vi "Elevator_Hopper_Manual.vi"(0 "Elevator_Control":T1={"DeviceStatus"={"status"=FALSE, "code"=0, "source"=""}, "Type"=enum."PWM", "PWM"={"PWM Channel"=enum."Invalid", "DeadBand"={"Name"="", "maxPositivePwm"=0, "minPositivePwm"=0, "centerPwm"=0, "maxNegativePwm"=0, "minNegativePwm"=0, "angularRange"=0}}, "CAN"={"Device Number"=0, "SetOutput VI Ref"=variant(enum8{"Percent VBus", "Current", "Speed", "Position", "Voltage"} enum."Percent VBus"), "GetOutput VI Ref"=variant(refnum<k1> refnum), "Enable VI Ref"=variant(dbl 12.0), "Disable VI Ref"=variant(enum8{"Percent VBus", "Speed", "Position", "Slave", "Unchanged / Invalid"} enum."Percent VBus"), "Data"=variant}, "Invert"=FALSE, "DIO PWM"={"PWM \"Enable\" Channel"=enum."Invalid", "DIOChannel"=enum."Invalid", "PWM Rate"=0.0}}, 1 "Hopper_Control":T1={"DeviceStatus"={"status"=FALSE, "code"=0, "source"=""}, "Type"=enum."PWM", "PWM"={"PWM Channel"=enum."Invalid", "DeadBand"={"Name"="", "maxPositivePwm"=0, "minPositivePwm"=0, "centerPwm"=0, "maxNegativePwm"=0, "minNegativePwm"=0, "angularRange"=0}}, "CAN"={"Device Number"=0, "SetOutput VI Ref"=variant(enum8{"Percent VBus", "Current", "Speed", "Position", "Voltage"} enum."Percent VBus"), "GetOutput VI Ref"=variant(refnum<k1> refnum), "Enable VI Ref"=variant(dbl 12.0), "Disable VI Ref"=variant(enum8{"Percent VBus", "Speed", "Position", "Slave", "Unchanged / Invalid"} enum."Percent VBus"), "Data"=variant}, "Invert"=FALSE, "DIO PWM"={"PWM \"Enable\" Channel"=enum."Invalid", "DIOChannel"=enum."Invalid", "PWM Rate"=0.0}}, 2 "Ball at Top":bool, 3 "Shoot":bool, 5 "Elevator_up":bool, 7 "Distance_to_target (in)":dbl, 9 "Elevator_Down":bool, 11 "Hopper Forwards":bool, 12 "Hopper Backwards":bool, 13 "Intake":bool) -> ()   [LabVIEW 2019]
uses:
  <vilib>/Rock Robotics/WPI/MotorControl/WPI_MotorControlDeviceRef.ctl
  <vilib>/Rock Robotics/WPI/MotorControl/WPI_MotorControlType.ctl
  <vilib>/Rock Robotics/SystemInterfaces/DIO/FPGA_DIOPWMChannel.ctl
  <vilib>/Rock Robotics/WPI/PWM/WPI_PWMDeadband.ctl
  <vilib>/Rock Robotics/SystemInterfaces/DIO/FPGA_DIOChannel.ctl
  ArgosLib/Signal Processing/TypeDefs/EdgeDetector_Type.ctl
  ArgosLib/ArgosLib.lvlib
panel:
  in  "Off":dbl[](array[numeric])=[0.0, 0.0, 0.0, 0.0, 0.0, 0.0]
  in  "Elevator Speeds down":dbl[](array[numeric])=[-0.8, -0.8, -0.8, -0.8, -0.8, -0.8]
  in  "Distances (in)":dbl[](array[numeric])=[51.5, 57.5, 120.0, 240.0, 360.0, 480.0]
  in  "Elevator Speeds":dbl[](array[numeric])=[1.0, 1.0, 0.6, 0.5, 0.4, 0.4]
  in  "Bakwards_Hopper":dbl=-0.5
  in  "Forwards_Hopper":dbl=0.7
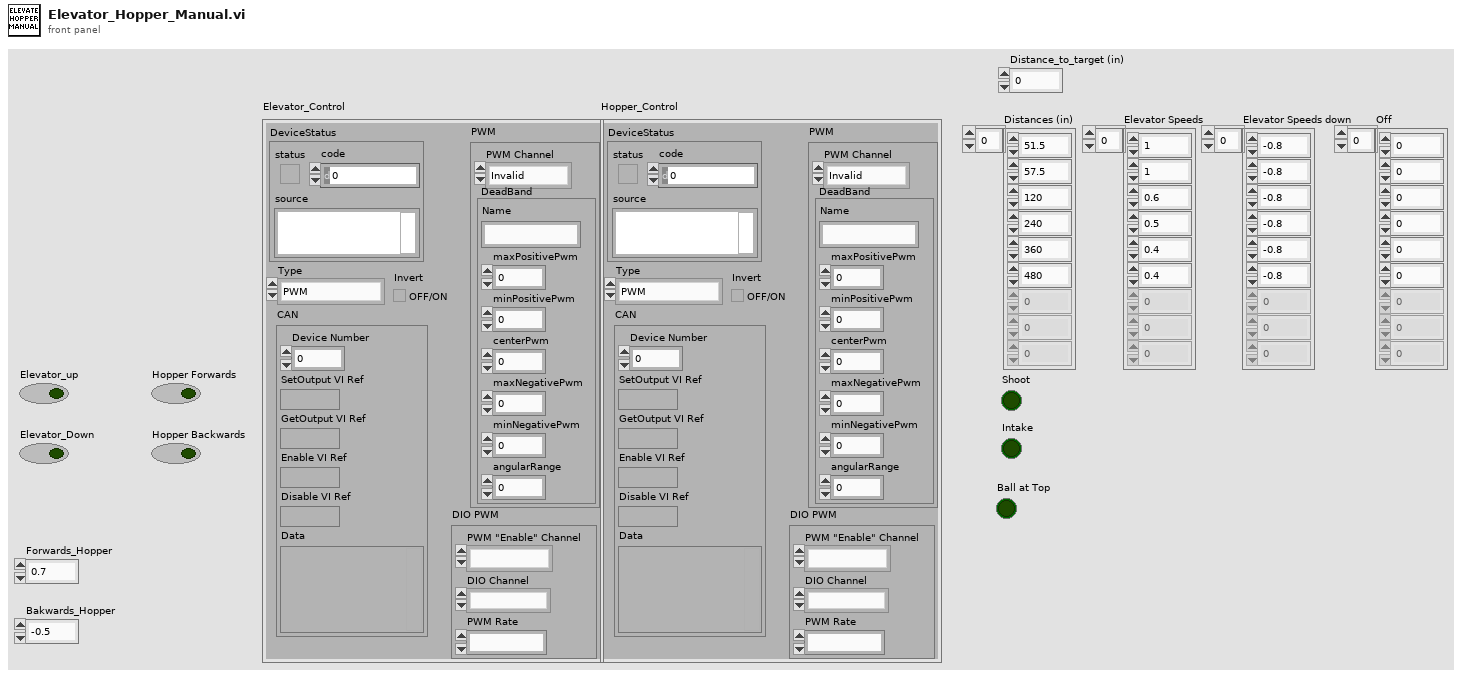
[diagram p1: front panel]
types:
  T1 = typedef "WPI_MotorControlDeviceRef.ctl" = cluster{"DeviceStatus":errorcluster, "Type":T2, "PWM":cluster{"PWM Channel":T3, "DeadBand":T4}, "CAN":cluster{"Device Number":u8, "SetOutput VI Ref":variant, "GetOutput VI Ref":variant, "Enable VI Ref":variant, "Disable VI Ref":variant, "Data":variant}, "Invert":bool, "DIO PWM":cluster{"PWM \"Enable\" Channel":T3, "DIOChannel":T5, "PWM Rate":dbl}}
  T2 = typedef "WPI_MotorControlType.ctl" = enum16{"PWM", "CAN", "DIO PWM"}
  T3 = typedef "FPGA_DIOPWMChannel.ctl" = enum8{"PWM 0", "PWM 1", "PWM 2", "PWM 3", "PWM 4", "PWM 5", "PWM 6", "PWM 7", "PWM 8", "PWM 9", "PWM MXP 0", "PWM MXP 1", "PWM MXP 2", "PWM MXP 3", "PWM MXP 4", "PWM MXP 5", "PWM MXP 6", "PWM MXP 7", "PWM MXP 8", "PWM MXP 9", "Invalid"}
  T4 = typedef "WPI_PWMDeadband.ctl" = cluster{"Name":string, "maxPositivePwm":i32, "minPositivePwm":i32, "centerPwm":i32, "maxNegativePwm":i32, "minNegativePwm":i32, "angularRange":u16}
  T5 = typedef "FPGA_DIOChannel.ctl" = enum8{"DIO 0", "DIO 1", "DIO 2", "DIO 3", "DIO 4", "DIO 5", "DIO 6", "DIO 7", "DIO 8", "DIO 9", "DIO MXP 0", "DIO MXP 1", "DIO MXP 2", "DIO MXP 3", "DIO MXP 4", "DIO MXP 5", "DIO MXP 6", "DIO MXP 7", "DIO MXP 8", "DIO MXP 9", "DIO MXP 10", "DIO MXP 11", "DIO MXP 12", "DIO MXP 13", "DIO MXP 14", "DIO MXP 15", "SPI Port CS1", "SPI Port CS2", "SPI Port CS3", "SPI Port MISO", "SPI Port MOSI", "Invalid"}
  T6 = typedef "ArgosLib.lvlib/EdgeDetector_Type.ctl" = enum16{"RisingEdge", "FallingEdge", "Both"}
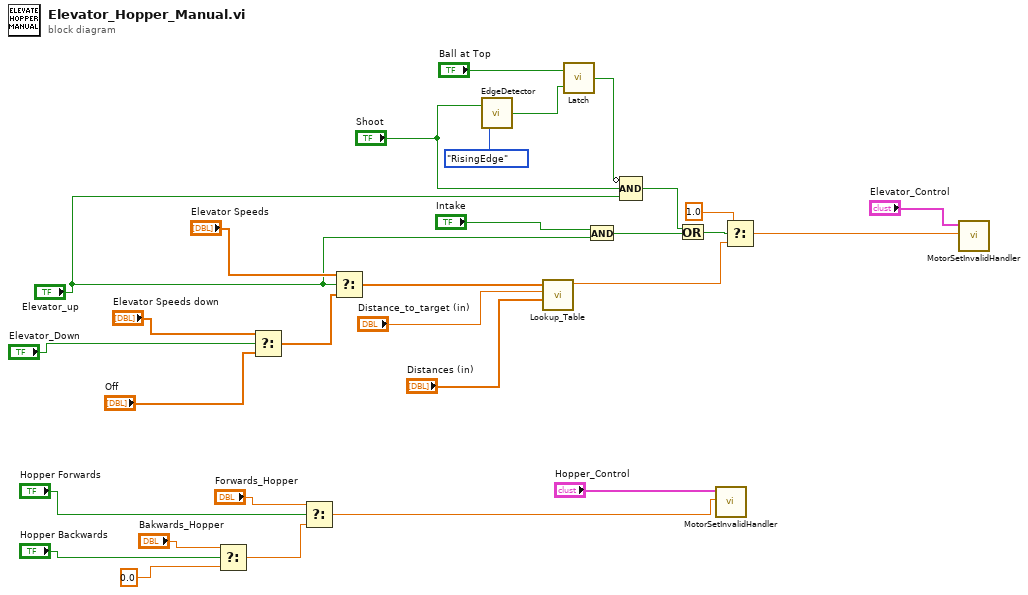
[diagram p0: block diagram]
diagram:
  n1 = Select(t="Bakwards_Hopper", s="Hopper Backwards", f=0.0 ("Stop_Hopper")) -> (s? t:f=w26:dbl)
  n2 = Select(t="Elevator Speeds down", s="Elevator_Down", f="Off") -> (s? t:f=w27:dbl[])
  n3 = Select(t="Forwards_Hopper", s="Hopper Forwards", f=w26) -> (s? t:f=w20:dbl)
  n4 = Select(t="Elevator Speeds", s="Elevator_up", f=w27) -> (s? t:f=w16:dbl[])
  n5 = call "EdgeDetector.vi"("DetectorType"=EdgeDetector_Type."RisingEdge", "Input"="Shoot") -> ("Edge"=w4:bool)
  n6 = call "Lookup_Table.vi"("Y_Array"=w16, "x_in"="Distance_to_target (in)", "X_Array"="Distances (in)") -> ("y_out"=w11:dbl)  [unwired: 6 in]
  n7 = call "Latch.vi"("Reset"=w4, "Input"="Ball at Top") -> ("LatchOut"=w2:bool)
  n8 = And(x="Intake", y="Elevator_up") -> (x .and. y?=w7:bool)
  n9 = Compound Arithmetic op=AND(invert w2, "Shoot", "Elevator_up") -> (w6:bool)
  n10 = Or(x=w6, y=w7) -> (x .or. y?=w8:bool)
  n11 = call "MotorSetInvalidHandler.vi"("Output"=w20, "MotorControlDevRef"="Hopper_Control") -> ()  [unwired: 7 in, 3 out]
  n12 = Select(t=1.0, s=w8, f=w11) -> (s? t:f=w10:dbl)
  n13 = call "MotorSetInvalidHandler.vi"("Output"=w10, "MotorControlDevRef"="Elevator_Control") -> ()  [unwired: 7 in, 3 out]
